vi "PathFile.vi"(11 "NameFile":string) -> (3 "stringNameFile":string)   [LabVIEW 2014]
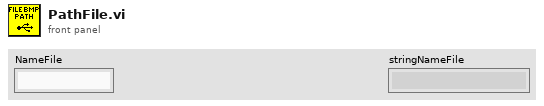
[diagram p1: front panel]
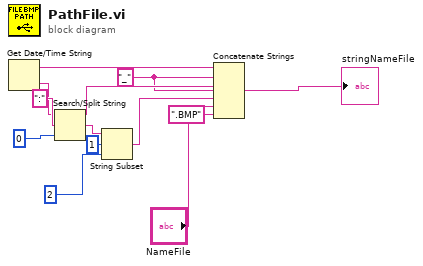
[diagram p0: block diagram]
diagram:
  w7 = "_"
  n1 = Get Date/Time String() -> (date string=w12:string, time string=w9:string)  [unwired: 3 in]
  n2 = Search/Split String(string=w9, search string/char (-)=":", offset (0)=0) -> (substring before match=w8:string, match + rest of string=w6:string)  [unwired: 1 out]
  n3 = String Subset(string=w6, offset (0)=1, length (rest)=2 ("length (rest)")) -> (substring=w3:string)
  n4 = Concatenate Strings(w12, w7, w8, w7, w3, "NameFile", ".BMP" ("string")) -> (→"stringNameFile":string)
